vi "Read IDs.vi"(8 "error in (no error)":errorcluster, 11 "System Actor in":refnum<class "System Actor.lvclass">) -> (0 "error out":errorcluster, 2 "IDs":i64[](array[numeric]), 3 "System Actor out":refnum<class "System Actor.lvclass">)   [LabVIEW 2024, in "System Actor.lvclass"]
uses:
  System Actor.lvclass
  System Actor.lvclass/System Actor.ctl
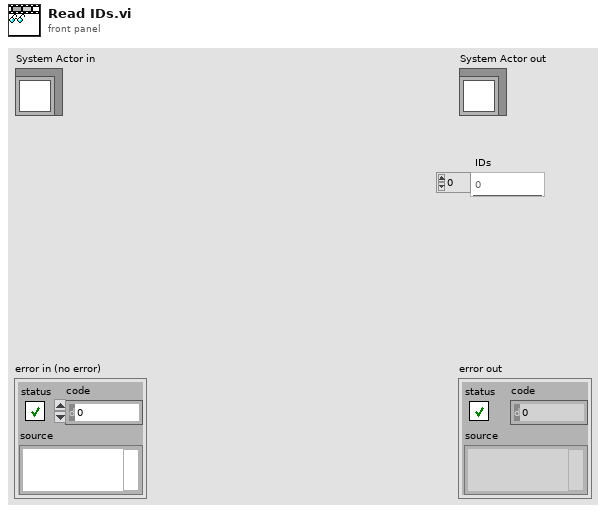
[diagram p1: front panel]
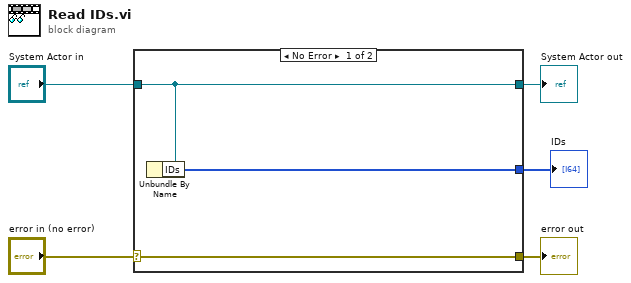
[diagram p0: block diagram]
diagram:
  n1 = case shown="No Error" "error in (no error)" {
    selector: "error in (no error)" -> [w8 w9]
    tunnel: [w8 w9] -> w4
    tunnel: [w7 w10] -> w2
    tunnel: "System Actor in" -> [w7 w10]
    tunnel: [w6 _] -> w1
    frame No Error {
      n2 = Unbundle By Name(w7) -> ("IDs"=w6:i64[])
    }
    frame Error {
    }
  }
  "error out" <- w4
  "System Actor out" <- w2
  "IDs" <- w1
